vi "Initialize Aquatrak.vi"(8 "error in (no error)":errorcluster) -> (0 "error out":errorcluster, 3 "Aquatrak COM Port":refnum<visa-resource-name>)   [LabVIEW 2019, in "Initialize.lvlib"]
uses:
  Initialize.lvlib
  <vilib>/Instr/_visa.llb/VISA Configure Serial Port (Instr).vi
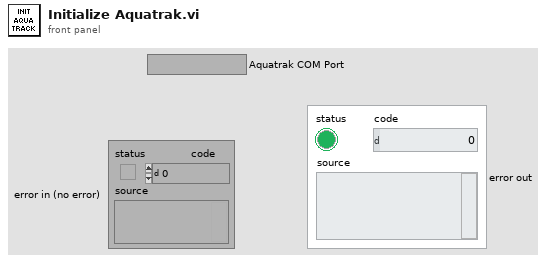
[diagram p1: front panel]
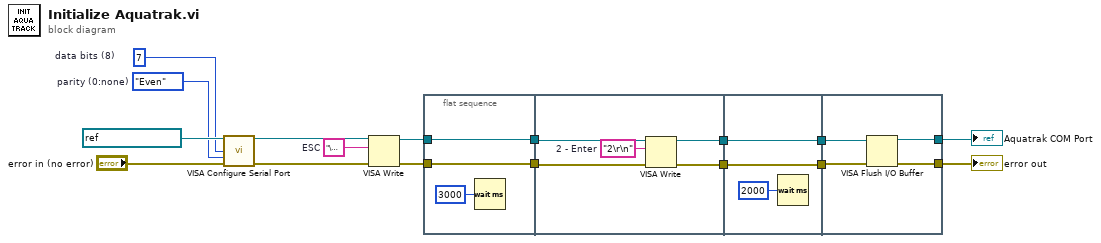
[diagram p0: block diagram]
diagram:
  w13 = "\u001b"  # ESC
  w14 = enum16{"None", "Odd", "Even", "Mark", "Space"}."Even"  # parity (0:none)
  w16 = u16 7  # data bits (8)
  n1 = call-poly "VISA Configure Serial Port"("VISA resource name"=refnum<visa-resource-name> "ASRL1::INSTR", "data bits (8)"=w16, "parity (0:none)"=w14, "error in (no error)"="error in (no error)") -> ("VISA resource name out"=w12:refnum<visa-resource-name>, "error out"=w11:errorcluster)  [unwired: 10 in]
  n2 = VISA Write(VISA resource name=w12, write buffer=w13, error in (no error)=w11) -> (VISA resource name out=w9:refnum<visa-resource-name>, error out=w10:errorcluster)  [unwired: 1 out]
  n3 = flat-sequence {
    tunnel: w10 -> [w19]
    tunnel: w9 -> [w20]
    tunnel: [w20] -> w8
    tunnel: [w19] -> w7
    tunnel: w8 -> [w24]
    tunnel: w7 -> [w23]
    tunnel: [w22] -> w4
    tunnel: [w21] -> w3
    tunnel: w4 -> [w27]
    tunnel: w3 -> [w26]
    tunnel: [w27] -> w2
    tunnel: [w26] -> w1
    tunnel: [w31] -> w5
    tunnel: [w32] -> w6
    tunnel: w2 -> [w30]
    tunnel: w1 -> [w29]
    frame #0 {
      n4 = Wait (ms)(milliseconds to wait=u32 3000) -> ()  [unwired: 1 out]
    }
    frame #1 {
      w25 = "2\r\n"  # 2 - Enter
      n5 = VISA Write(VISA resource name=w24, write buffer=w25, error in (no error)=w23) -> (VISA resource name out=w22:refnum<visa-resource-name>, error out=w21:errorcluster)  [unwired: 1 out]
    }
    frame #2 {
      n6 = Wait (ms)(milliseconds to wait=u32 2000) -> ()  [unwired: 1 out]
    }
    frame #3 {
      n7 = VISA Flush I/O Buffer(VISA resource name=w30, error in (no error)=w29) -> (VISA resource name out=w32:refnum<visa-resource-name>, error out=w31:errorcluster)  [unwired: 1 in]
    }
  }
  "Aquatrak COM Port" <- w6
  "error out" <- w5
